vi "Main_modular.vi"   [LabVIEW 2021]
uses:
  Main_modular_state.ctl
  QueueEnum.ctl
types:
  T1 = typedef "Main_modular_state.ctl" = enum16{"Init", "Run", "Exit"}
  T2 = enum32{"Invalid", "Standard", "Closed", "Hidden", "Minimized", "Maximized"}
  T3 = typedef "QueueEnum.ctl" = enum16{"Obtain Queue", "Get Queue Ref", "Flush Queue", "Release Queue"}
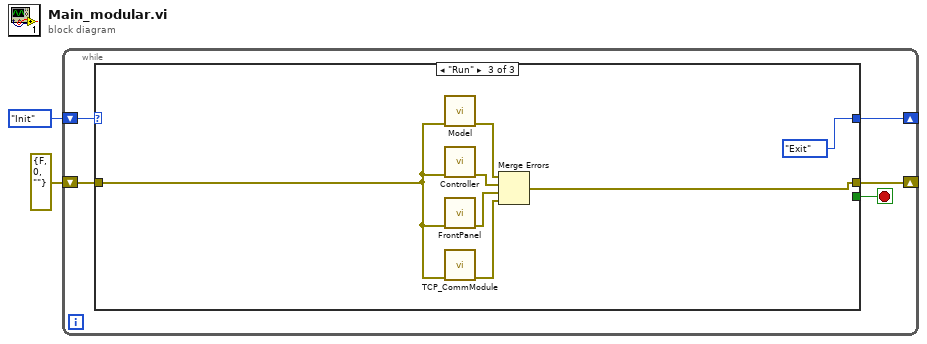
[diagram p0: block diagram]
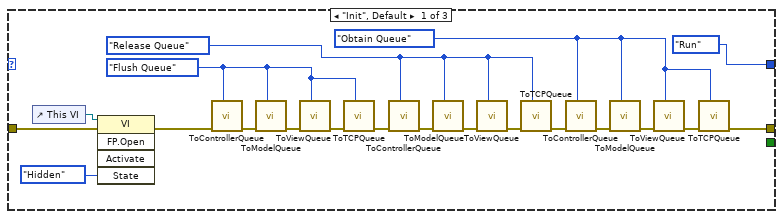
[diagram p2: hidden frame]
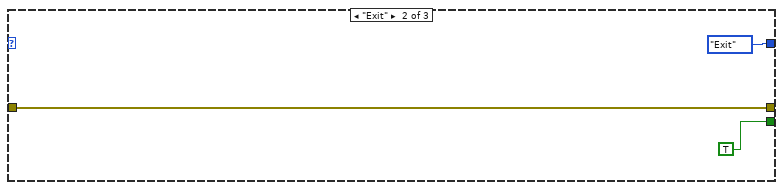
[diagram p3: hidden frame]
diagram:
  n1 = while {
    shift-right: [w5] -> _
    shift-left: errorcluster {"status"=FALSE, "code"=0, "source"=""} ("error constant") -> [w6]
    shift-right: [w4] -> _
    shift-left: Main_modular_state."Init" -> [w7]
    stop <- w3 stop-if-true
    n2 = case shown="\"Run\"" w7 {
      tunnel: w6 -> [w25 w29 w33]
      tunnel: [w8 w29 w34] -> w5
      tunnel: [Main_modular_state."Run" Main_modular_state."Exit" Main_modular_state."Exit"] -> w4
      tunnel: [_ TRUE _] -> w3
      frame "Init", Default {
        w11 = QueueEnum."Obtain Queue"
        w15 = QueueEnum."Release Queue"
        w20 = QueueEnum."Flush Queue"
        n3 = control-ref of="This VI"() -> (w27:refnum<vi>)
        n4 = invoke class="VI" method="FP.Open"(reference=w27, error in=w25, "State"=T2."Hidden") -> (error out=w21:errorcluster)  [unwired: 2 in, 4 out]
        n5 = call "ToControllerQueue.vi"("Enum"=w20, "error in (no error)"=w21) -> ("error out"=w24:errorcluster)  [unwired: 8 in, 1 out]
        n6 = call "ToModelQueue.vi"("Enum"=w20, "error in (no error)"=w24) -> ("error out"=w23:errorcluster)  [unwired: 8 in, 1 out]
        n7 = call "ToViewQueue.vi"("Enum"=w20, "error in (no error)"=w23) -> ("error out"=w22:errorcluster)  [unwired: 8 in, 1 out]
        n8 = call "ToTCPQueue.vi"("Enum"=w20, "error in (no error)"=w22) -> ("error out"=w10:errorcluster)  [unwired: 8 in, 1 out]
        n9 = call "ToControllerQueue.vi"("Enum"=w15, "error in (no error)"=w10) -> ("error out"=w18:errorcluster)  [unwired: 8 in, 1 out]
        n10 = call "ToModelQueue.vi"("Enum"=w15, "error in (no error)"=w18) -> ("error out"=w17:errorcluster)  [unwired: 8 in, 1 out]
        n11 = call "ToViewQueue.vi"("Enum"=w15, "error in (no error)"=w17) -> ("error out"=w16:errorcluster)  [unwired: 8 in, 1 out]
        n12 = call "ToTCPQueue.vi"("Enum"=w15, "error in (no error)"=w16) -> ("error out"=w9:errorcluster)  [unwired: 8 in, 1 out]
        n13 = call "ToControllerQueue.vi"("Enum"=w11, "error in (no error)"=w9) -> ("error out"=w14:errorcluster)  [unwired: 8 in, 1 out]
        n14 = call "ToModelQueue.vi"("Enum"=w11, "error in (no error)"=w14) -> ("error out"=w13:errorcluster)  [unwired: 8 in, 1 out]
        n15 = call "ToViewQueue.vi"("Enum"=w11, "error in (no error)"=w13) -> ("error out"=w12:errorcluster)  [unwired: 8 in, 1 out]
        n16 = call "ToTCPQueue.vi"("Enum"=w11, "error in (no error)"=w12) -> ("error out"=w8:errorcluster)  [unwired: 8 in, 1 out]
      }
      frame "Exit" {
      }
      frame "Run" {
        n17 = call "Model.vi"("error in (no error)"=w33) -> ("error out"=w32:errorcluster)  [unwired: 10 in]
        n18 = call "Controller.vi"("error in (no error)"=w33) -> ("error out"=w31:errorcluster)  [unwired: 10 in]
        n19 = call "FrontPanel.vi"("error in (no error)"=w33) -> ("error out"=w35:errorcluster)  [unwired: 10 in]
        n20 = call "TCP_CommModule.vi"("error in (no error)"=w33) -> ("error out"=w36:errorcluster)  [unwired: 10 in]
        n21 = Merge Errors(w32, w31, w35, w36) -> (w34:errorcluster)
      }
    }
  }
